vi "Read Session Out.vi"(8 "error in (no error)":errorcluster, 11 "Webcam in":refnum<class "Webcam.lvclass">) -> (0 "error out":errorcluster, 2 "IMAQdx Session":T1, 3 "Webcam out":refnum<class "Webcam.lvclass">)   [LabVIEW 2020, in "Webcam.lvclass"]
uses:
  Webcam.lvclass
  <vilib>/userDefined/High Color/IMAQdx.ctl
  Webcam.lvclass/Webcam.ctl
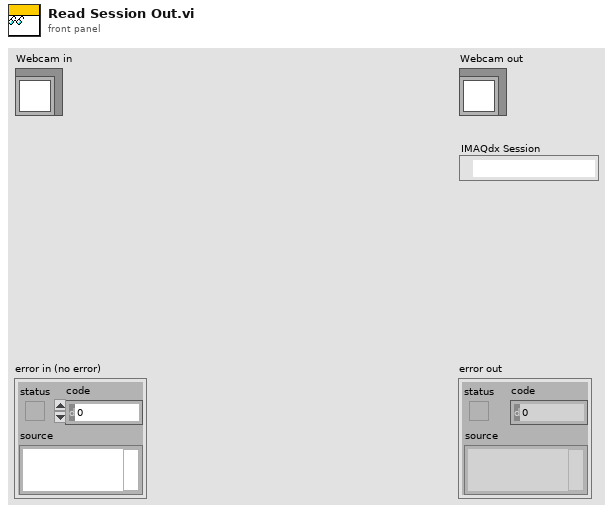
[diagram p1: front panel]
types:
  T1 = typedef "IMAQdx.ctl" = refnum<k21>
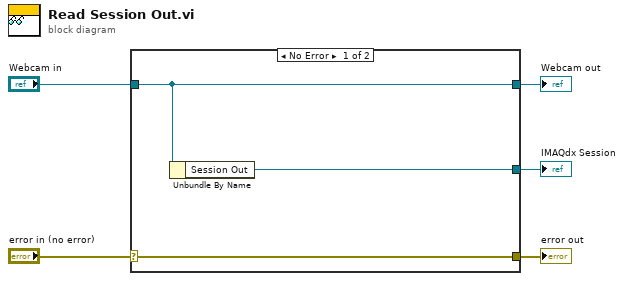
[diagram p0: block diagram]
diagram:
  n1 = case shown="No Error" "error in (no error)" {
    selector: "error in (no error)" -> [w8 w9]
    tunnel: [w8 w9] -> w4
    tunnel: [w7 w10] -> w2
    tunnel: "Webcam in" -> [w7 w10]
    tunnel: [w6 _] -> w1
    frame No Error {
      n2 = Unbundle By Name(w7) -> ("Session Out"=w6:T1)
    }
    frame Error {
    }
  }
  "error out" <- w4
  "Webcam out" <- w2
  "IMAQdx Session" <- w1
